vi "Robot Global Data.vi"() -> ()   [LabVIEW 2014]
doc: "This global VI can contain as many global variables as you need. Place a control on the panel, give it a good name. To read or write to it from a VI, drag the icon to the diagram of that VI. You can also drag from the project. Click on the node to change which global you access. You shouldn't have multiple locations writing to a global or it will cause a race-condition."
uses:
  <vilib>/Rock Robotics/WPI/Camera/WPI_CameraImageSize.ctl
  <vilib>/Rock Robotics/WPI/DriverStation/WPI_DriverStationRobotMode2.ctl
panel:
  in  "SlowDrive":bool
  in  "ResetSensors":bool
  in  "ArmOpen":bool
  in  "LiftDown":bool
  out "ZAxis":dbl
  in  "IntakeBoth":bool
  in  "IntakeRight":bool
  in  "IntakeLeft":bool
  in  "LiftUp":bool
  in  "ArmClose":bool
  out "YAxis":dbl
  out "XAxis":dbl
  in  "Clockwise":bool
  in  "CounterClockwise":bool
  out "AngularAccel":dbl
  out "RotateVal":dbl
  out "Rotating":bool
  out "Error":dbl
  in  "DesiredHeading":dbl
  out "CurrentHeading":dbl
  in  "Robot Mode 2":T1
  in  "image size 2":T2=enum."320x240"
  in  "Enable Vision 2":bool
  in  "Robot Mode":T1
  in  "image size":T2=enum."320x240"
  in  "Enable Vision":bool
  # "current angle the front of the \nrobot is facing, relative to the \nbeginning of the match"
  # "the angle the robot's face should \nbe at, relative to the start of the match."
  # "whether or not the \nrobot is rotating"
  # "The error between CurrentHeading \nand DesiredHeading to calculate rotation"
  # "speed the robot is rotating. -1 to 1\n(1 being full speed clockwise)"
  # "the rate at which the robot\n is changing angle."
  # "controls/indicates the direction the \nrobot is rotating"
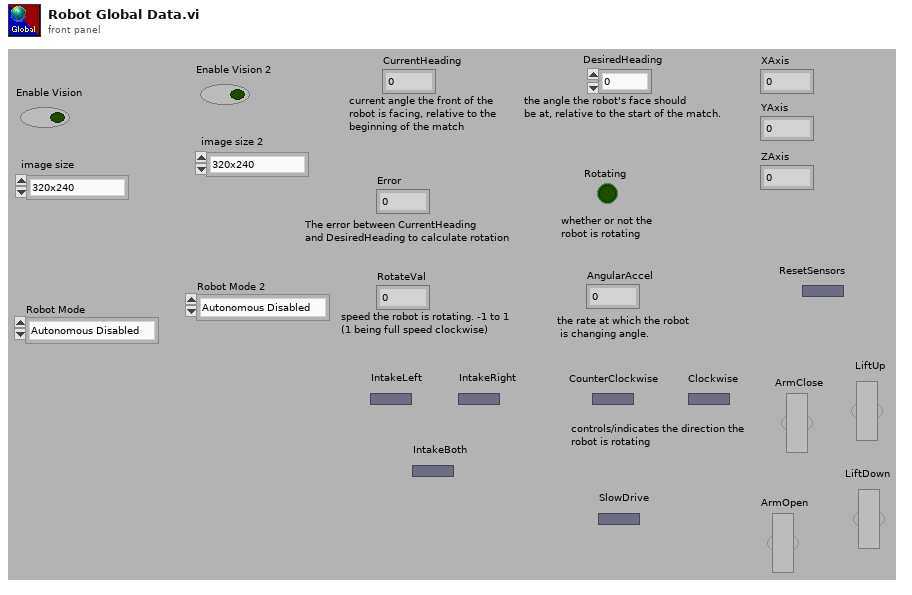
[diagram p1: front panel]
types:
  T1 = typedef "WPI_DriverStationRobotMode2.ctl" = enum16{"Autonomous Disabled", "Autonomous Enabled", "Teleop Disabled", "Teleop Enabled", "Disconnected", "Finish", "Test Disabled", "Test Enabled", "Emergency Stopped"}
  T2 = typedef "WPI_CameraImageSize.ctl" = enum16{"640x480", "320x240", "160x120", "Custom"}
diagram:
